vi "Convert to i64 Timestamp.vi"(2 "Packet Header":T1) -> (4 "Timestamp (ns)":i64)   [LabVIEW 2021, in "pcap_Parse_Build_CIF.lvclass"]
uses:
  pcap_Parse_Build_CIF.lvclass
  pcap_Parse_Build_CIF.lvclass/pcap_Parse_Build_CIF.ctl
  Typedef/Packet Header.ctl
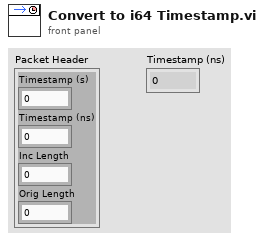
[diagram p1: front panel]
types:
  T1 = typedef "pcap_Parse_Build_CIF.lvclass/Packet Header.ctl" = cluster{"Timestamp (s)":u32, "Timestamp (ns)":u32, "Inc Length":u32, "Orig Length":u32}
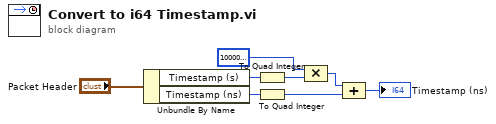
[diagram p0: block diagram]
diagram:
  n1 = Unbundle By Name("Packet Header") -> ("Timestamp (s)"=w7:u32, "Timestamp (ns)"=w4:u32)
  n2 = To Quad Integer(1:w7) -> (0:w5:i64)
  n3 = To Quad Integer(1:w4) -> (0:w3:i64)
  n4 = Compound Arithmetic op=MULTIPLY(i64 1000000000 ("value"), w5) -> (w2:i64)
  n5 = Compound Arithmetic op=ADD(w2, w3) -> (→"Timestamp (ns)":i64)
